vi "night time stamp.vi"(8 "error in (no error)":errorcluster) -> (0 "error out":errorcluster, 2 "date time rec":T1)   [LabVIEW 2018]
uses:
  <vilib>/Utility/miscctls.llb/LVDateTimeRec.ctl
panel:
  in  "zero":T1
  in  "1 day":T1
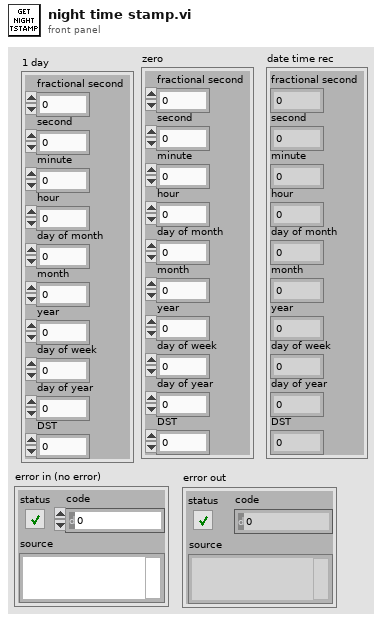
[diagram p1: front panel]
types:
  T1 = typedef "LVDateTimeRec.ctl" = cluster{"fractional second":dbl, "second":i32, "minute":i32, "hour":i32, "day of month":i32, "month":i32, "year":i32, "day of week":i32, "day of year":i32, "DST":i32}
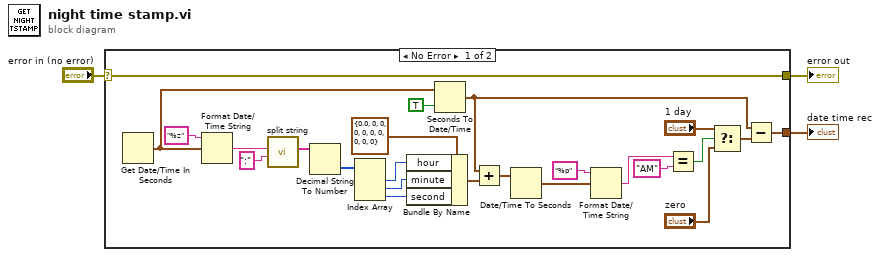
[diagram p0: block diagram]
diagram:
  n1 = case shown="No Error" "error in (no error)" {
    selector: "error in (no error)" -> [w27 w28]
    tunnel: [w27 w28] -> w2
    tunnel: [w7 _] -> w1
    frame No Error {
      n2 = Get Date/Time In Seconds() -> (seconds since 1Jan1904=w17:timestamp)
      n3 = Format Date/Time String(time format string (%c)="%z", seconds (now)=w17) -> (date/time string=w24:string)  [unwired: 1 in]
      n4 = call "split string.vi"("search string"=":", "String"=w24) -> ("strings array"=w22:string[])  [unwired: 8 in, 1 out]
      n5 = Decimal String To Number(string=w22) -> (number=w21:i32[])  [unwired: 2 in, 1 out]
      n6 = Index Array(array=w21) -> (element #1=w20:i32, element #2=w19:i32, element #3=w18:i32)  [unwired: 3 in]
      n7 = Bundle By Name(cluster=T1 {"fractional second"=0.0, "second"=0, "minute"=0, "hour"=0, "day of month"=0, "month"=0, "year"=0, "day of week"=0, "day of year"=0, "DST"=0} ("date time rec 2"), "hour"=w20, "minute"=w19, "second"=w18) -> (w15:T1)
      n8 = Seconds To Date/Time(time stamp (now)=w17, to UTC (F)=TRUE) -> (date time rec=w8:T1)
      n9 = Add(x=w8, y=w15) -> (x+y=w4:T1)
      n10 = Date/Time To Seconds(2:w4) -> (0:w14:timestamp)  [unwired: 1 in]
      n11 = Format Date/Time String(time format string (%c)="%p", seconds (now)=w14) -> (date/time string=w9:string)  [unwired: 1 in]
      n12 = Equal?(x=w9, y="AM") -> (x = y?=w11:bool)
      n13 = Select(t="1 day", s=w11, f="zero") -> (s? t:f=w12:T1)
      n14 = Subtract(x=w8, y=w12) -> (x-y=w7:T1)
    }
    frame Error {
    }
  }
  "error out" <- w2
  "date time rec" <- w1
